vi "PhaseToPOW.vi"(1 "Phase":dbl) -> (0 "POW [14bit]":u16)   [LabVIEW 2013]
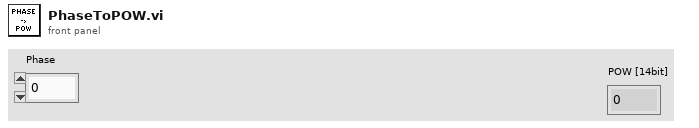
[diagram p1: front panel]
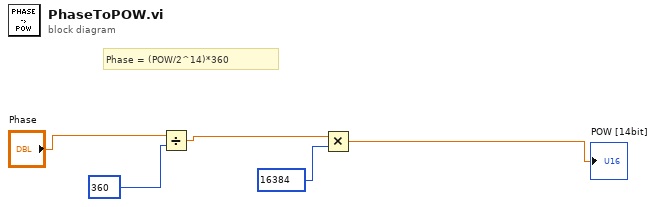
[diagram p0: block diagram]
diagram:
  # "Phase = (POW/2^14)*360"
  n1 = Divide(x="Phase", y=360) -> (x/y=w3:dbl)
  n2 = Multiply(x=w3, y=u64 16384) -> (x*y=→"POW [14bit]":dbl)
